vi "TestPowerMeter.vi"() -> ()   [LabVIEW 2018]
panel:
  in  "stop":bool
  out "Measurement":sgl
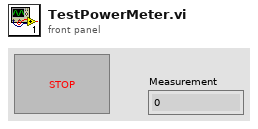
[diagram p1: front panel]
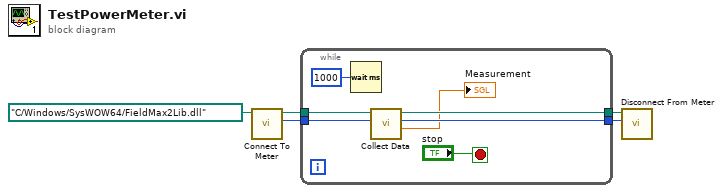
[diagram p0: block diagram]
diagram:
  n1 = call "Connect To Meter.vi"("Location of FieldMax2Lib.dll in"=path "C:/Windows/SysWOW64/FieldMax2Lib.dll") -> ("Meter ID out"=w2:i32, "Location of FieldMax2Lib.dll out"=w1:path)  [unwired: 6 in, 1 out]
  n2 = while {
    tunnel: w2 -> [w12]
    tunnel: w1 -> [w11]
    tunnel: [w10] -> w4
    tunnel: [w9] -> w3
    stop <- "stop" stop-if-true
    n3 = Wait (ms)(milliseconds to wait=u32 1000) -> ()  [unwired: 1 out]
    n4 = call <instrlib>:"Collect Data.vi"("Location of FieldMax2Lib.dll in"=w11, "Meter ID in"=w12) -> ("Location of FieldMax2Lib.dll out"=w10:path, "Meter ID out"=w9:i32, "Measurement"=→"Measurement":sgl)  [unwired: 5 in, 1 out]
  }
  n5 = call <instrlib>:"Disconnect From Meter.vi"("Location of FieldMax2Lib.dll in"=w4, "Meter ID in"=w3) -> ()  [unwired: 7 in, 2 out]
